vi "Set Spool.vi"(7 "framebuffersize":i32, 8 "error in (no error)":errorcluster, 9 "path":string, 10 "method":i32, 11 "active":i32) -> (0 "error out":errorcluster, 1 "path out":string, 3 "function return":u32)   [LabVIEW 2014, in "atmcd32d.lvlib"]
doc: "unsigned int WINAPI SetSpool(int active, int method, char * path, int framebuffersize);"
uses:
  atmcd32d.lvlib
  atmcd32d.dll
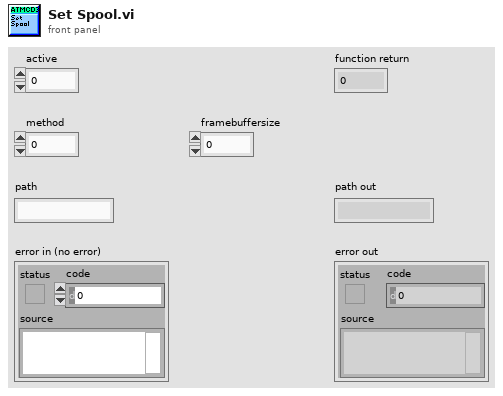
[diagram p1: front panel]
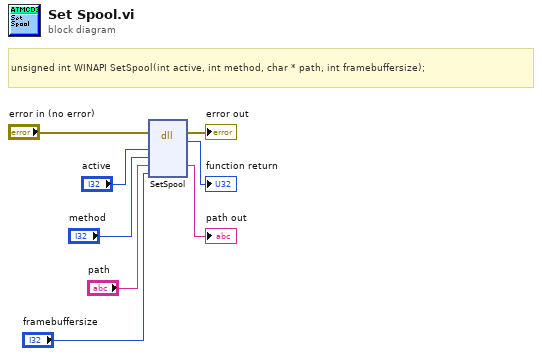
[diagram p0: block diagram]
diagram:
  # "unsigned int WINAPI SetSpool(int active, int method, char * path, int framebuffersize);"
  n1 = dll-call lib="C:/Users/Bakir/Documents/Lambda2-Testing/lib/Andorlib/atmcd32d.*" fn="SetSpool"(error in="error in (no error)", "active"="active", "method"="method", "path"="path", "framebuffersize"="framebuffersize") -> (error out=→"error out":errorcluster, →"function return":u32, "path"=→"path out":string)  [unwired: 5 in, 1 out]
